vi "ConvertTimestampToDateTime.vi"(11 "Timestamp":dbl format="%<%I:%M:%S%3u %p\n%m/%d/%Y>T") -> (2 "Time string":string, 3 "date string":string)   [LabVIEW 2018, in "Library-DataConvert.lvlib"]
uses:
  Library-DataConvert.lvlib
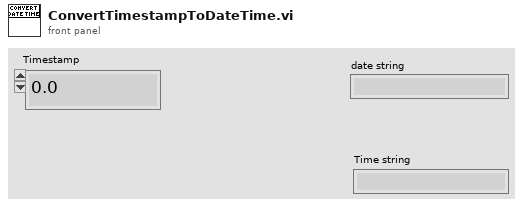
[diagram p1: front panel]
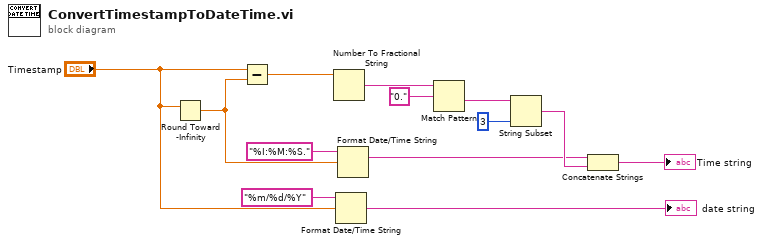
[diagram p0: block diagram]
diagram:
  n1 = Round Toward -Infinity(1:"Timestamp") -> (0:w2:dbl)
  n2 = Subtract(x="Timestamp", y=w2) -> (x-y=w10:dbl)
  n3 = Number To Fractional String(number=w10) -> (F-format string=w8:string)  [unwired: 3 in]
  n4 = Format Date/Time String(time format string (%c)="%m/%d/%Y", seconds (now)="Timestamp") -> (date/time string=→"date string":string)  [unwired: 1 in]
  n5 = Format Date/Time String(time format string (%c)="%I:%M:%S.", seconds (now)=w2) -> (date/time string=w4:string)  [unwired: 1 in]
  n6 = Match Pattern(string=w8, regular expression="0.") -> (after substring=w7:string)  [unwired: 1 in, 3 out]
  n7 = String Subset(string=w7, length (rest)=3 ("length")) -> (substring=w5:string)  [unwired: 1 in]
  n8 = Concatenate Strings(w4, w5) -> (→"Time string":string)
